vi "Build Send Method.vi"(6 "Wiring Spec":T2, 8 "error in (no error)":errorcluster, 9 "AF Library FQN":string, 10 "References":T1, 11 "Send VI":refnum<vi>) -> (0 "error out":errorcluster)   [LabVIEW 2023, in "Message Maker.lvclass"]
doc: "Build The send vi for the new message\n\nAuthor: Derek Trepanier\nCopyright: MGI 2015"
uses:
  Message Maker.lvclass
  Wiring Spec.ctl
  Connector Pane Position.ctl
  Scripting Refs.ctl
  <vilib>/Utility/traverseref.llb/TRef TravTarget.ctl
  <vilib>/Utility/miscctls.llb/LVPointTypeDef.ctl
  <vilib>/Utility/traverseref.llb/VI Scripting - Traverse.lvlib
  <vilib>/LabVIEW Icon API/LabVIEW Icon API.lvlib
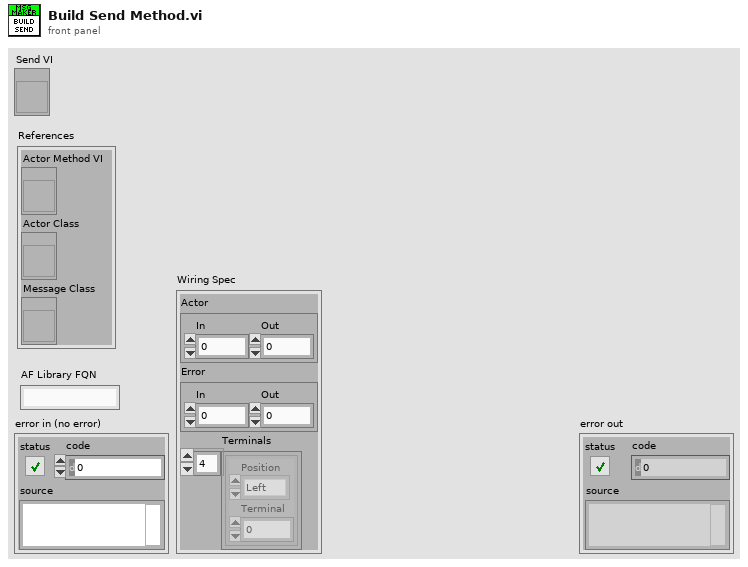
[diagram p1: front panel]
types:
  T1 = typedef "Message Maker.lvclass/Scripting Refs.ctl" = cluster{"Actor Method VI":refnum<vi>, "Actor Class":refnum<vi>, "Message Class":refnum<vi>}
  T2 = typedef "Message Maker.lvclass/Wiring Spec.ctl" = cluster{"Actor":cluster{"In":i32, "Out":i32}, "Error":cluster{"In":i32, "Out":i32}, "Terminals":cluster{"Position":T3, "Terminal":i32}[]}
  T3 = typedef "Message Maker.lvclass/Connector Pane Position.ctl" = enum16{"Left", "Top", "Bottom", "Right"}
  T4 = cluster{"Left":cluster{"Position":i16, "Index":i32}[], "Bottom":cluster{"Position":i16, "Index":i32}[], "Right":cluster{"Position":i16, "Index":i32}[], "Top":cluster{"Position":i16, "Index":i32}[]}
  T5 = enum16{"Replace Classes", "Configure Connector", "Add FP Controls", "Wire Bundle", "Set Icon and Desc", "Build BD"}
  T6 = typedef "TRef TravTarget.ctl" = enum16{"FP", "BD", "Other"}
  T7 = typedef "LVPointTypeDef.ctl" = cluster{"Horizontal":i16, "Vertical":i16}
  T8 = typedef "LVRectTypeDef.ctl" = cluster{"Left":i16, "Top":i16, "Right":i16, "Bottom":i16}
  T9 = enum16{"Invalid Wire Rule", "Required", "Recommended", "Optional", "Dynamic Dispatch"}[]
  T10 = cluster{cluster{"Position":i16, "Index":i32}[]}[]
  T11 = enum16{"Invalid Wire Rule", "Required", "Recommended", "Optional", "Dynamic Dispatch"}
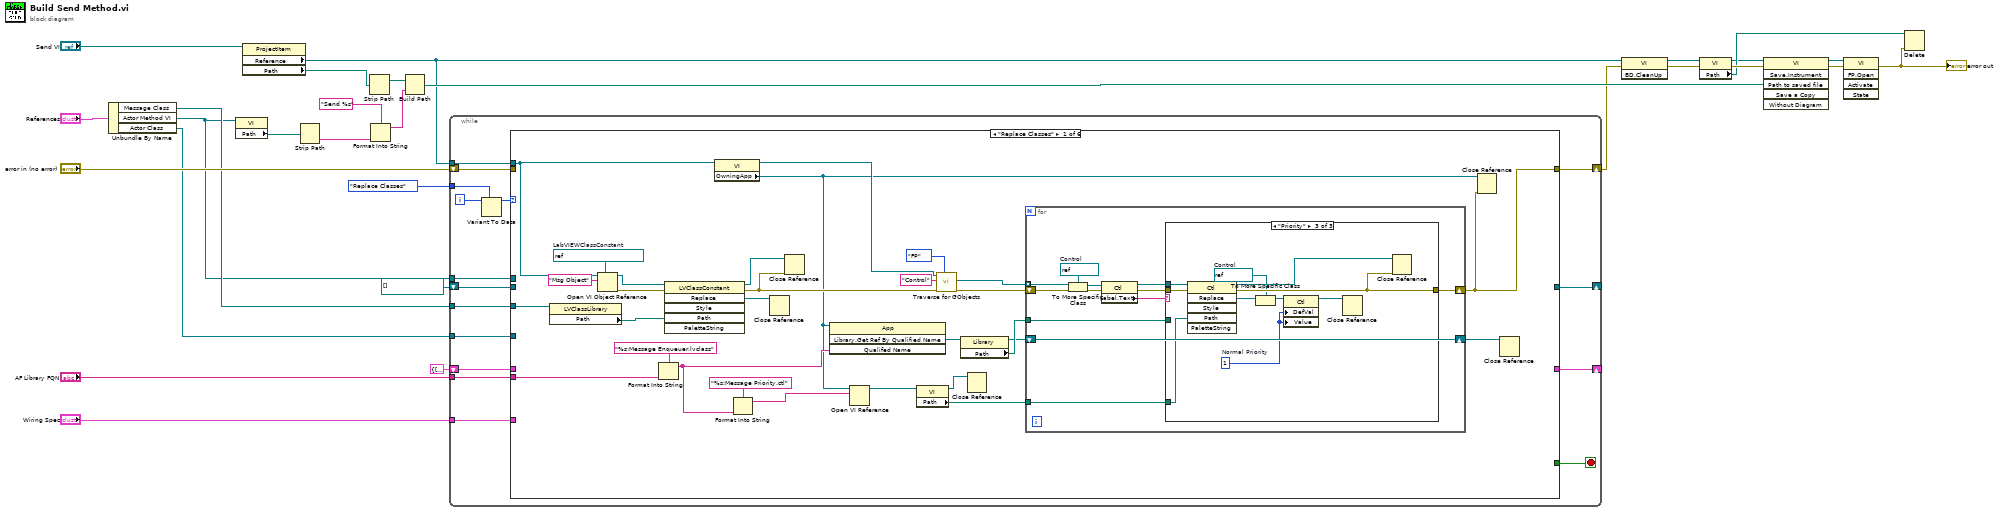
[diagram p0: block diagram]
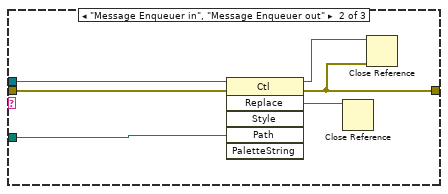
[diagram p3: hidden frame]
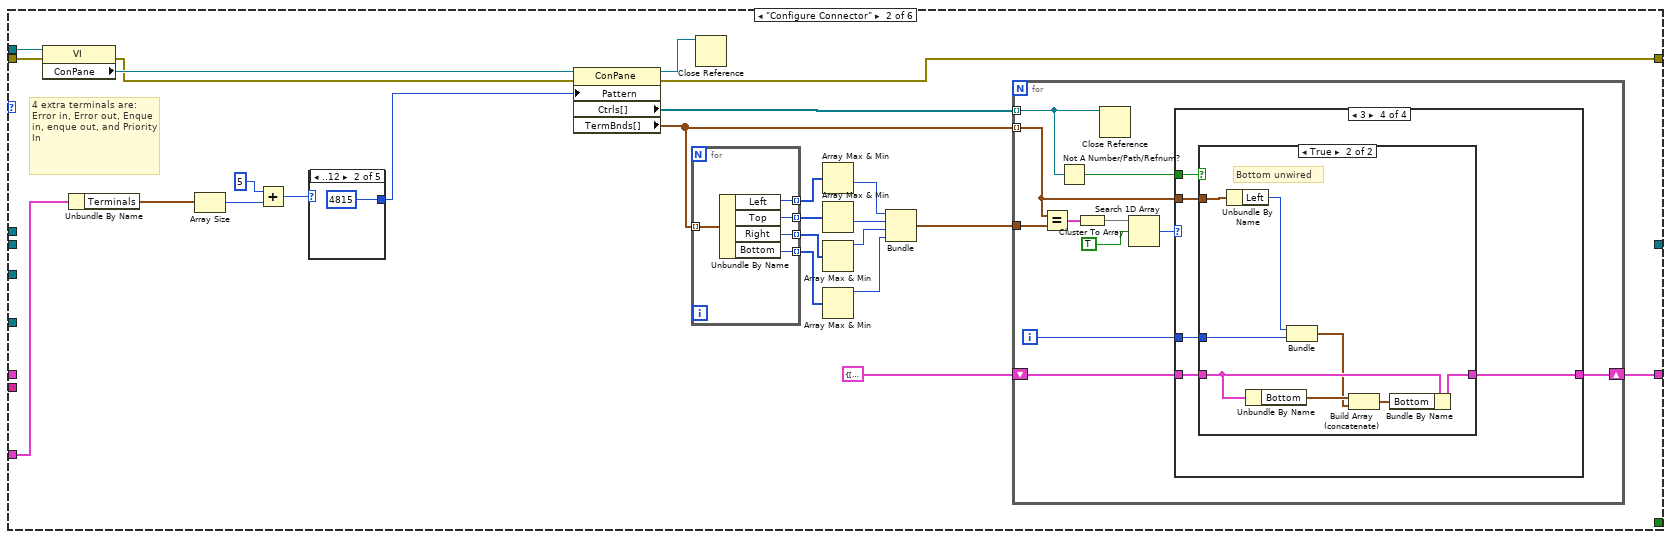
[diagram p4: hidden frame]
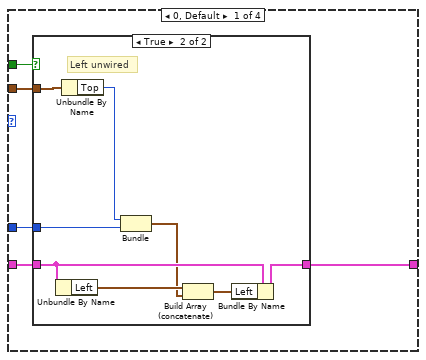
[diagram p5: hidden frame]
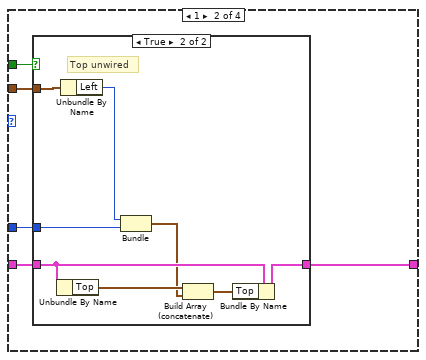
[diagram p7: hidden frame]
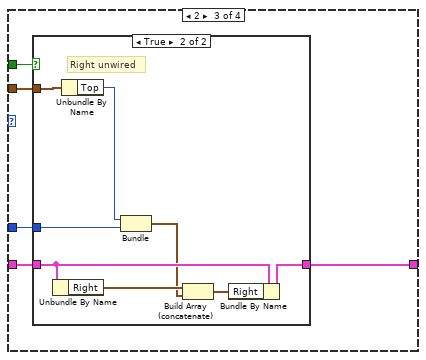
[diagram p9: hidden frame]
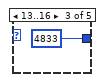
[diagram p13: hidden frame]
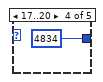
[diagram p14: hidden frame]
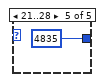
[diagram p15: hidden frame]
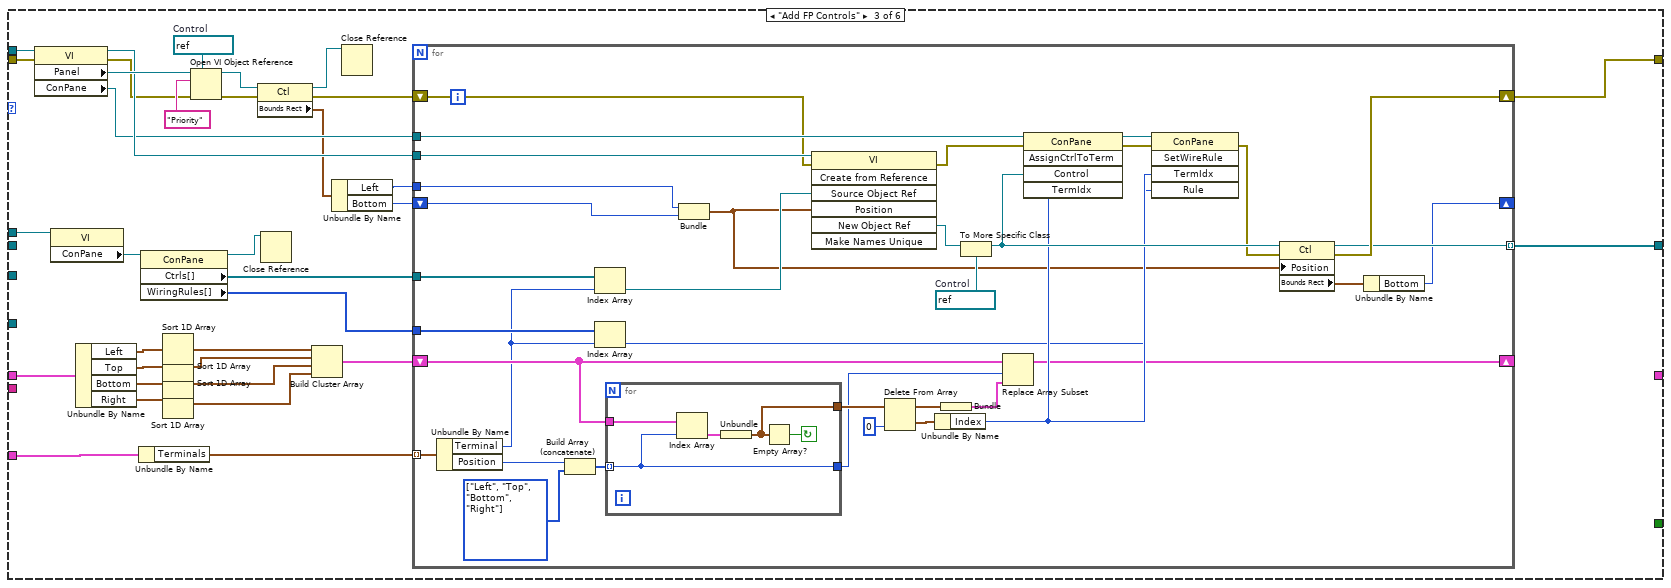
[diagram p16: hidden frame]
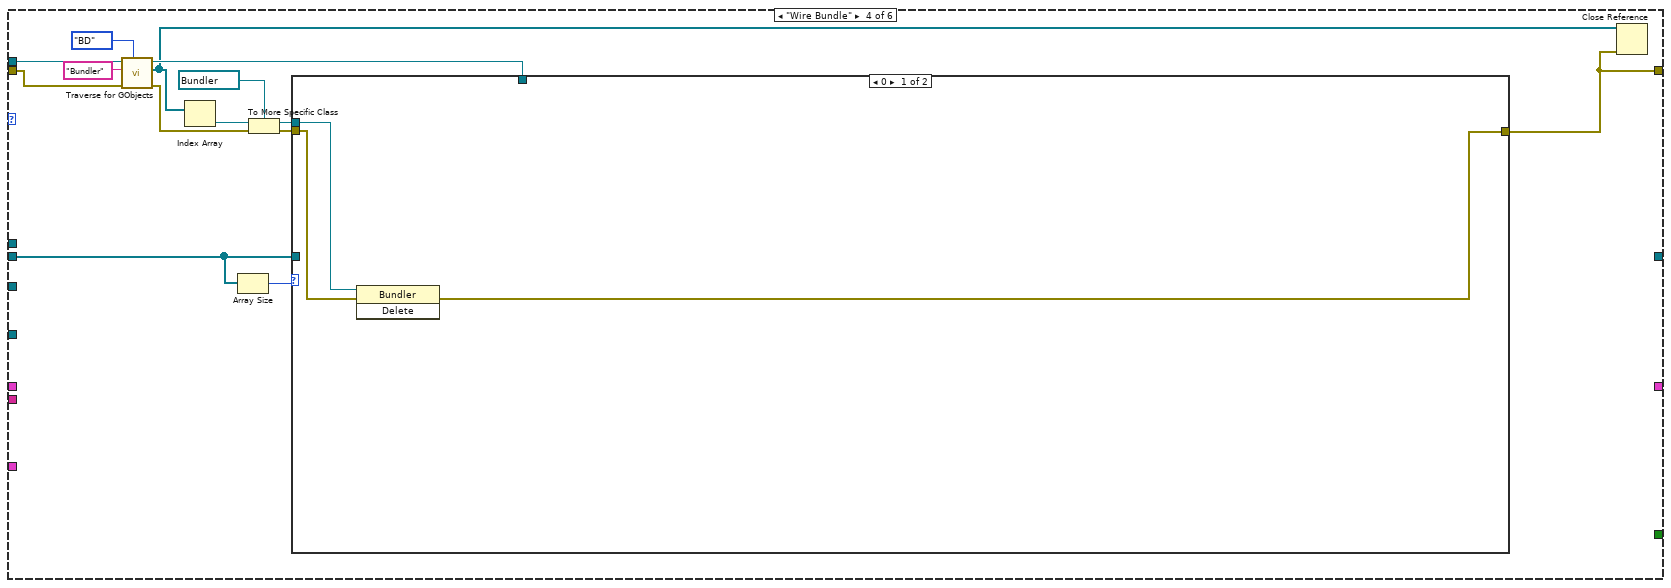
[diagram p17: hidden frame]
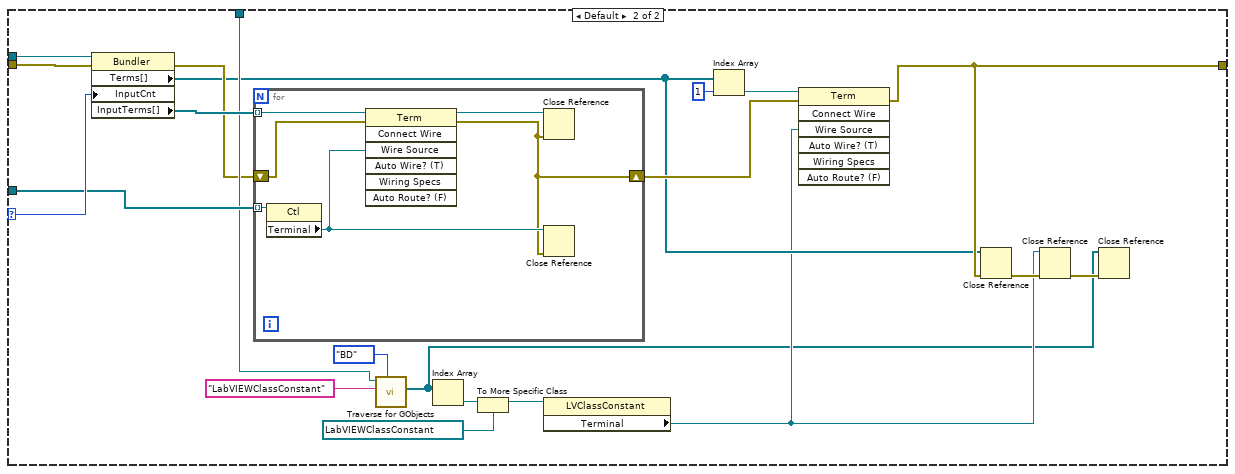
[diagram p18: hidden frame]
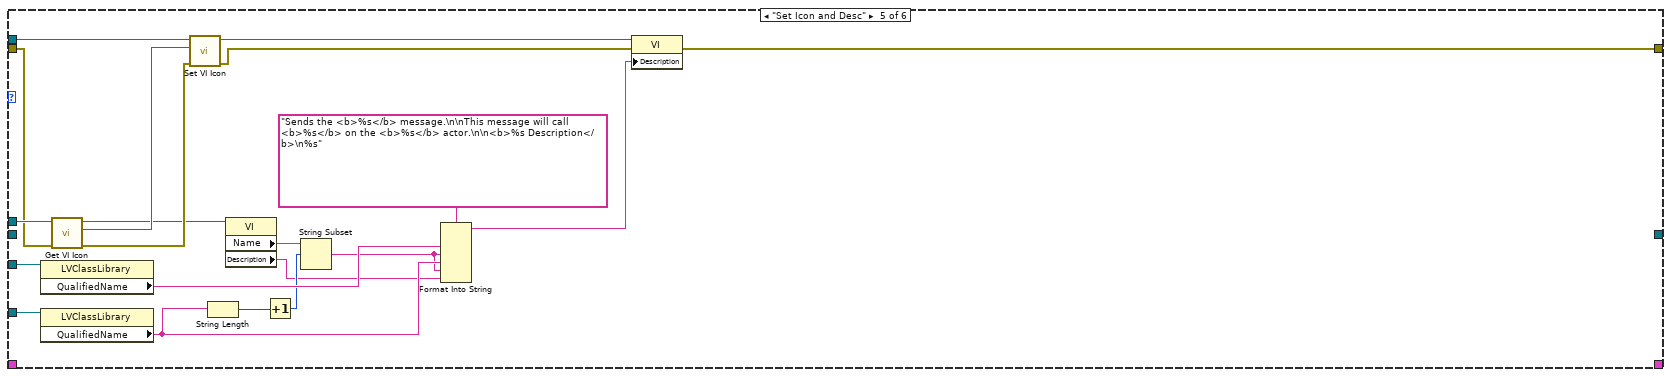
[diagram p19: hidden frame]
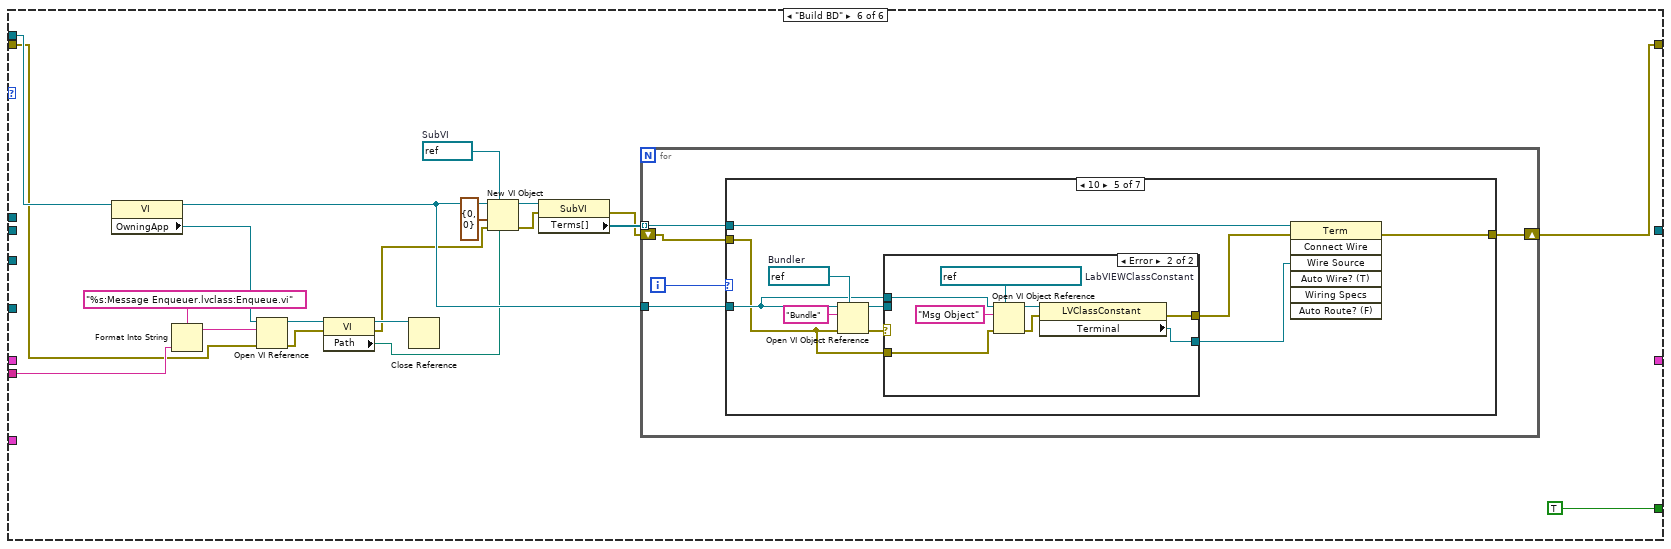
[diagram p20: hidden frame]
diagram:
  n1 = Unbundle By Name("References") -> ("Message Class"=w10:refnum<vi>, "Actor Method VI"=w5:refnum<vi>, "Actor Class"=w9:refnum<vi>)
  n2 = property class="VI"(reference=w5) -> ("Path"=w4:path)  [unwired: 1 in, 2 out]
  n3 = property class="ProjectItem"(reference="Send VI") -> ("Reference"=w19:refnum<vi>, "Path"=w25:path)  [unwired: 1 in, 2 out]
  n4 = Strip Path(path=w4) -> (name=w3:string)  [unwired: 1 out]
  n5 = Strip Path(path=w25) -> (stripped path=w24:path)  [unwired: 1 out]
  n6 = Format Into String(format string="Send %s", w3) -> (resulting string=w23:string)  [unwired: 2 in, 1 out]
  n7 = Build Path(base path=w24, name or relative path=w23) -> (appended path=w22:path)
  n8 = while {
    tunnel: T5."Replace Classes" -> [w44]
    tunnel: "Wiring Spec" -> [w41]
    tunnel: w19 -> [w40]
    tunnel: w5 -> [w39]
    shift-right: [w36] -> w17
    shift-left: "error in (no error)" -> [w37]
    shift-right: [w35] -> _
    shift-left: T4 {"Left"=[], "Bottom"=[], "Right"=[], "Top"=[]} -> [w34]
    shift-right: [w33] -> _
    shift-left: refnum<vi>[] [] -> [w32]
    tunnel: w10 -> [w31]
    tunnel: w9 -> [w30]
    tunnel: "AF Library FQN" -> [w29]
    i -> [w43]
    stop <- w38 stop-if-true
    n9 = Variant To Data(type=w44, Variant=w43) -> (data=w42:T5)  [unwired: 1 in, 1 out]
    n10 = case shown="\"Replace Classes\"" w42 {
      tunnel: w41 -> [_ w127 w228 _ _ _]
      tunnel: w40 -> [w62 w126 w237 w278 w340 w356]
      tunnel: w39 -> [_ _ w230 _ w341 _]
      tunnel: [_ _ _ _ _ TRUE] -> w38
      tunnel: w37 -> [_ w121 w223 w291 w324 w344]
      tunnel: [w46 w119 w220 w279 w322 w347] -> w36
      tunnel: [_ w103 _ _ _ _] -> w35
      tunnel: w34 -> [_ _ w219 _ _ _]
      tunnel: [_ _ w207 _ _ _] -> w33
      tunnel: w32 -> [_ _ _ w286 _ _]
      tunnel: w31 -> [w71 _ _ _ w333 _]
      tunnel: w30 -> [_ _ _ _ w331 _]
      tunnel: w29 -> [w48 _ _ _ _ w349]
      frame "Replace Classes" {
        w68 = refnum<vi> refnum  # LabVIEWClassConstant
        n11 = property class="LVClassLibrary"(reference=w71) -> ("Path"=w73:path)  [unwired: 1 in, 2 out]
        n12 = Open VI Object Reference(7:w68, 10:"Msg Object" ("name/order"), 11:w62) -> (0:w70:errorcluster, 3:w69:refnum<vi>)  [unwired: 1 in]
        n13 = Format Into String(format string="%s:Message Enqueuer.lvclass", w48) -> (resulting string=w49:string)  [unwired: 2 in, 1 out]
        n14 = invoke class="LVClassConstant" method="Replace"(reference=w69, error in=w70, "Path"=w73) -> (reference out=w67:refnum<vi>, error out=w63:errorcluster, "Replace"=w72:refnum<vi>)  [unwired: 3 in, 3 out]
        n15 = property class="VI"(reference=w62) -> (reference out=w59:refnum<vi>, "OwningApp"=w45:refnum<vi>)  [unwired: 1 in, 1 out]
        n16 = Format Into String(format string="%s:Message Priority.ctl", w49) -> (resulting string=w53:string)  [unwired: 2 in, 1 out]
        n17 = Close Reference(reference=w72) -> ()  [unwired: 1 in, 1 out]
        n18 = Close Reference(reference=w67, error in (no error)=w63) -> ()  [unwired: 1 out]
        n19 = invoke class="App" method="Library.Get Ref By Qualified Name"(reference=w45, "Qualifed Name"=w49) -> ("Library.Get Ref By Qualified Name"=w58:refnum<vi>)  [unwired: 2 in, 3 out]
        n20 = Open VI Reference(application reference (local)=w45, vi path=w53) -> (vi reference=w52:refnum<vi>)  [unwired: 4 in, 1 out]
        n21 = property class="VI"(reference=w52) -> (reference out=w47:refnum<vi>, "Path"=w51:path)  [unwired: 1 in, 1 out]
        n22 = call <vilib>:"Traverse for GObjects.vi"("Traverse Target"=TRef_TravTarget."FP", "error in (no error)"=w63, "Class Name"="Control" ("name/order"), "VI Refnum"=w59) -> ("error out"=w64:errorcluster, "References"=w60:refnum<vi>[])  [unwired: 4 in, 2 out]
        n23 = property class="Library"(reference=w58) -> (reference out=w56:refnum<vi>, "Path"=w57:path)  [unwired: 1 in, 1 out]
        n24 = Close Reference(reference=w47) -> ()  [unwired: 1 in, 1 out]
        n25 = for {
          tunnel: w60 -> [w78] mode=indexing
          tunnel: w57 -> [w84]
          shift-right: [w83] -> w46
          shift-left: w64 -> [w85]
          shift-right: [w82] -> w55
          shift-left: w56 -> [w82]
          tunnel: w51 -> [w74]
          w76 = refnum<vi> refnum  # Control
          n26 = To More Specific Class(target class=w76, reference=w78, error in=w85) -> (specific class reference=w77:refnum<vi>, error out=w79:errorcluster)
          n27 = property class="Ctl"(reference=w77, error in=w79) -> (reference out=w80:refnum<vi>, error out=w81:errorcluster, "Label.Text"=w75:string)
          n28 = case shown="\"Priority\"" w75 {
            tunnel: w84 -> [_ w90 _]
            tunnel: [w86 w89 w100] -> w83
            tunnel: w81 -> [w86 w88 w99]
            tunnel: w80 -> [_ w87 w98]
            tunnel: w74 -> [_ _ w97]
            frame "False", Default {
            }
            frame "Message Enqueuer in", "Message Enqueuer out" {
              n29 = invoke class="Ctl" method="Replace"(reference=w87, error in=w88, "Path"=w90) -> (reference out=w92:refnum<vi>, error out=w89:errorcluster, "Replace"=w91:refnum<vi>)  [unwired: 3 in, 3 out]
              n30 = Close Reference(reference=w91) -> ()  [unwired: 1 in, 1 out]
              n31 = Close Reference(reference=w92, error in (no error)=w89) -> ()  [unwired: 1 out]
            }
            frame "Priority" {
              w93 = 1  # Normal Priority
              w94 = refnum<vi> refnum  # Control
              n32 = invoke class="Ctl" method="Replace"(reference=w98, error in=w99, "Path"=w97) -> (reference out=w102:refnum<vi>, error out=w100:errorcluster, "Replace"=w101:refnum<vi>)  [unwired: 3 in, 3 out]
              n33 = To More Specific Class(target class=w94, reference=w101) -> (specific class reference=w95:refnum<vi>)  [unwired: 1 in, 1 out]
              n34 = property class="Ctl"(reference=w95, "DefVal"=w93, "Value"=w93) -> (reference out=w96:refnum<vi>)  [unwired: 1 in, 1 out]
              n35 = Close Reference(reference=w96) -> ()  [unwired: 1 in, 1 out]
              n36 = Close Reference(reference=w102, error in (no error)=w100) -> ()  [unwired: 1 out]
            }
          }
        }
        n37 = Close Reference(reference=w45, error in (no error)=w46) -> ()  [unwired: 1 out]
        n38 = Close Reference(reference=w55) -> ()  [unwired: 1 in, 1 out]
      }
      frame "Configure Connector" {
        # "4 extra terminals are:\nError in, Error out, Enque in, enque out, and Priority In"
        n39 = property class="VI"(reference=w126, error in=w121) -> (error out=w120:errorcluster, "ConPane"=w125:refnum<vi>)  [unwired: 1 out]
        n40 = Unbundle By Name(w127) -> ("Terminals"=w124:cluster{"Position":T3, "Terminal":i32}[])
        n41 = Array Size(array=w124) -> (size(s)=w118:i32)
        n42 = Add(x=5, y=w118) -> (x+y=w116:i32)
        n43 = case shown="..12" w116 {
          tunnel: [_ u32 4815 ("Pattern") u32 4833 ("Pattern") u32 4834 ("Pattern") u32 4835 ("Pattern")] -> w122
          frame Default {
          }
          frame ..12 {
          }
          frame 13..16 {
          }
          frame 17..20 {
          }
          frame 21..28 {
          }
        }
        n44 = property class="ConPane"(reference=w125, error in=w120, "Pattern"=w122) -> (reference out=w123:refnum<vi>, error out=w119:errorcluster, "Ctrls[]"=w109:refnum<vi>[], "TermBnds[]"=w107:T8[])
        n45 = for {
          tunnel: w107 -> [w199] mode=indexing
          tunnel: [w198] -> w115 mode=indexing
          tunnel: [w197] -> w114 mode=indexing
          tunnel: [w196] -> w113 mode=indexing
          tunnel: [w195] -> w112 mode=indexing
          n46 = Unbundle By Name(w199) -> ("Left"=w198:i16, "Top"=w197:i16, "Right"=w196:i16, "Bottom"=w195:i16)
        }
        n47 = Close Reference(reference=w123) -> ()  [unwired: 1 in, 1 out]
        n48 = Array Max & Min(array=w115) -> (min value=w106:i16)  [unwired: 3 out]
        n49 = Array Max & Min(array=w114) -> (min value=w105:i16)  [unwired: 3 out]
        n50 = Array Max & Min(array=w113) -> (max value=w111:i16)  [unwired: 3 out]
        n51 = Array Max & Min(array=w112) -> (max value=w110:i16)  [unwired: 3 out]
        n52 = Bundle(w106, w105, w111, w110) -> (w108:cluster{i16, i16, i16, i16})  [unwired: 1 in]
        n53 = for {
          tunnel: w109 -> [w133] mode=indexing
          tunnel: w108 -> [w138]
          tunnel: w107 -> [w130] mode=indexing
          shift-right: [w129] -> w103
          shift-left: T4 {"Left"=[], "Bottom"=[], "Right"=[], "Top"=[]} -> [w131]
          i -> [w128]
          n54 = Equal?(x=w130, y=w138) -> (x = y?=w137:cluster{bool, bool, bool, bool})
          n55 = Not A Number/Path/Refnum?(number/path/refnum=w133) -> (NaN/Path/Refnum?=w132:bool)
          n56 = Cluster To Array(cluster=w137) -> (array=w136:bool[])
          n57 = Close Reference(reference=w133) -> ()  [unwired: 1 in, 1 out]
          n58 = Search 1D Array(1D array=w136, element=TRUE) -> (index of element=w134:i32)  [unwired: 1 in]
          n59 = case shown="3" w134 {
            tunnel: w132 -> [w143 w157 w171 w185]
            tunnel: w131 -> [w142 w156 w170 w184]
            tunnel: w130 -> [w141 w155 w169 w183]
            tunnel: [w140 w154 w168 w182] -> w129
            tunnel: w128 -> [w139 w153 w167 w181]
            frame 0, Default {
              n60 = case shown="True" w143 {
                tunnel: w142 -> [w144 w151]
                tunnel: w141 -> [_ w152]
                tunnel: [w144 w148] -> w140
                tunnel: w139 -> [_ w149]
                frame False {
                }
                frame True {
                  # "Left unwired"
                  n61 = Unbundle By Name(w151) -> ("Left"=w147:cluster{"Position":i16, "Index":i32}[])
                  n62 = Unbundle By Name(w152) -> ("Top"=w150:i16)
                  n63 = Bundle("Top"=w150, w149) -> (w145:cluster{"Top":i16, i32})  [unwired: 1 in]
                  n64 = Build Array (concatenate)(w147, w145) -> (w146:cluster{"Top":i16, "Index":i32}[])
                  n65 = Bundle By Name(cluster=w151, "Left"=w146) -> (w148:T4)
                }
              }
            }
            frame 1 {
              n66 = case shown="True" w157 {
                tunnel: w156 -> [w158 w165]
                tunnel: w155 -> [_ w166]
                tunnel: [w158 w162] -> w154
                tunnel: w153 -> [_ w163]
                frame False {
                }
                frame True {
                  # "Top unwired"
                  n67 = Unbundle By Name(w165) -> ("Top"=w161:cluster{"Position":i16, "Index":i32}[])
                  n68 = Unbundle By Name(w166) -> ("Left"=w164:i16)
                  n69 = Bundle("Left"=w164, w163) -> (w159:cluster{"Left":i16, i32})  [unwired: 1 in]
                  n70 = Build Array (concatenate)(w161, w159) -> (w160:cluster{"Left":i16, "Index":i32}[])
                  n71 = Bundle By Name(cluster=w165, "Top"=w160) -> (w162:T4)
                }
              }
            }
            frame 2 {
              n72 = case shown="True" w171 {
                tunnel: w170 -> [w172 w179]
                tunnel: w169 -> [_ w180]
                tunnel: [w172 w176] -> w168
                tunnel: w167 -> [_ w177]
                frame False {
                }
                frame True {
                  # "Right unwired"
                  n73 = Unbundle By Name(w179) -> ("Right"=w175:cluster{"Position":i16, "Index":i32}[])
                  n74 = Unbundle By Name(w180) -> ("Top"=w178:i16)
                  n75 = Bundle("Top"=w178, w177) -> (w173:cluster{"Top":i16, i32})  [unwired: 1 in]
                  n76 = Build Array (concatenate)(w175, w173) -> (w174:cluster{"Top":i16, "Index":i32}[])
                  n77 = Bundle By Name(cluster=w179, "Right"=w174) -> (w176:T4)
                }
              }
            }
            frame 3 {
              n78 = case shown="True" w185 {
                tunnel: w184 -> [w186 w193]
                tunnel: w183 -> [_ w194]
                tunnel: [w186 w190] -> w182
                tunnel: w181 -> [_ w191]
                frame False {
                }
                frame True {
                  # "Bottom unwired"
                  n79 = Unbundle By Name(w194) -> ("Left"=w192:i16)
                  n80 = Unbundle By Name(w193) -> ("Bottom"=w189:cluster{"Position":i16, "Index":i32}[])
                  n81 = Bundle("Left"=w192, w191) -> (w187:cluster{"Left":i16, i32})  [unwired: 1 in]
                  n82 = Build Array (concatenate)(w189, w187) -> (w188:cluster{"Left":i16, "Index":i32}[])
                  n83 = Bundle By Name(cluster=w193, "Bottom"=w188) -> (w190:T4)
                }
              }
            }
          }
        }
      }
      frame "Add FP Controls" {
        w236 = refnum<vi> refnum  # Control
        n84 = property class="VI"(reference=w237, error in=w223) -> (reference out=w225:refnum<vi>, error out=w222:errorcluster, "Panel"=w234:refnum<vi>, "ConPane"=w224:refnum<vi>)
        n85 = property class="VI"(reference=w230) -> ("ConPane"=w229:refnum<vi>)  [unwired: 1 in, 2 out]
        n86 = Unbundle By Name(w219) -> ("Left"=w218:cluster{"Position":i16, "Index":i32}[], "Top"=w217:cluster{"Position":i16, "Index":i32}[], "Bottom"=w215:cluster{"Position":i16, "Index":i32}[], "Right"=w216:cluster{"Position":i16, "Index":i32}[])
        n87 = Unbundle By Name(w228) -> ("Terminals"=w226:cluster{"Position":T3, "Terminal":i32}[])
        n88 = property class="ConPane"(reference=w229) -> (reference out=w209:refnum<vi>, "Ctrls[]"=w227:refnum<vi>[], "WiringRules[]"=w210:T9)  [unwired: 1 in, 1 out]
        n89 = Sort 1D Array(array=w218) -> (sorted array=w214:cluster{"Position":i16, "Index":i32}[])
        n90 = Sort 1D Array(array=w217) -> (sorted array=w208:cluster{"Position":i16, "Index":i32}[])
        n91 = Sort 1D Array(array=w215) -> (sorted array=w213:cluster{"Position":i16, "Index":i32}[])
        n92 = Sort 1D Array(array=w216) -> (sorted array=w212:cluster{"Position":i16, "Index":i32}[])
        n93 = Open VI Object Reference(7:w236, 8:w222, 10:"Priority" ("name/order"), 11:w234) -> (0:w231:errorcluster, 3:w233:refnum<vi>)
        n94 = property class="Ctl"(reference=w233, error in=w231) -> (reference out=w232:refnum<vi>, error out=w221:errorcluster, "Bounds Rect"=w206:T8)
        n95 = Close Reference(reference=w209) -> ()  [unwired: 1 in, 1 out]
        n96 = Build Cluster Array(w214, w208, w213, w212) -> (w211:T10)
        n97 = Unbundle By Name(w206) -> ("Left"=w205:i16, "Bottom"=w204:i16)
        n98 = Close Reference(reference=w232) -> ()  [unwired: 1 in, 1 out]
        n99 = for {
          tunnel: w227 -> [w272]
          tunnel: w226 -> [w264] mode=indexing
          tunnel: w225 -> [w271]
          tunnel: w224 -> [w270]
          shift-right: [w265] -> w220
          shift-left: w221 -> [w267]
          shift-right: [w249] -> _
          shift-left: w211 -> [w257]
          tunnel: w210 -> [w248]
          tunnel: [w245] -> w207 mode=indexing
          tunnel: w205 -> [w239]
          shift-right: [w240] -> _
          shift-left: w204 -> [w238]
          w262 = T3[] [enum."Left", enum."Top", enum."Bottom", enum."Right"] items=["Left", "Top", "Bottom", "Right"] ("appended array")
          w269 = refnum<vi> refnum  # Control
          n100 = Unbundle By Name(w264) -> ("Terminal"=w246:i32, "Position"=w263:T3)
          n101 = Build Array (concatenate)(w263, w262) -> (w261:T3[])
          n102 = Index Array(array=w272, index=w246) -> (element=w243:refnum<vi>)
          n103 = Index Array(array=w248, index=w246) -> (element=w247:T11)
          n104 = for {
            tunnel: w257 -> [w277]
            tunnel: w261 -> [w274] mode=indexing
            tunnel: [w274] -> w255
            tunnel: [w273] -> w260
            stop <- w275 continue-if-true
            n105 = Index Array(array=w277, index=w274) -> (element=w276:cluster{cluster{"Position":i16, "Index":i32}[]})
            n106 = Unbundle(w276) -> (w273:cluster{"Position":i16, "Index":i32}[])
            n107 = Empty Array?(array=w273) -> (empty?=w275:bool)
          }
          n108 = Bundle("Left"=w239, "Bottom"=w238) -> (w242:cluster{"Left":i16, "Bottom":i16})  [unwired: 1 in]
          n109 = invoke class="VI" method="Create from Reference"(reference=w271, error in=w267, "Source Object Ref"=w243, "Position"=w242) -> (error out=w266:errorcluster, "New Object Ref"=w244:refnum<vi>)  [unwired: 3 in, 5 out]
          n110 = Delete From Array(array=w260, index=0) -> (deleted portion=w254:cluster{"Position":i16, "Index":i32}, array with subset deleted=w258:cluster{"Position":i16, "Index":i32}[])  [unwired: 1 in]
          n111 = Unbundle By Name(w254) -> ("Index"=w250:i32)
          n112 = Bundle(w258) -> (w256:cluster{cluster{"Position":i16, "Index":i32}[]})  [unwired: 1 in]
          n113 = To More Specific Class(target class=w269, reference=w244) -> (specific class reference=w268:refnum<vi>)  [unwired: 1 in, 1 out]
          n114 = Replace Array Subset(array=w257, new element=w256, index=w255) -> (w249:T10)
          n115 = invoke class="ConPane" method="AssignCtrlToTerm"(reference=w270, error in=w266, "Control"=w268, "TermIdx"=w250) -> (reference out=w253:refnum<vi>, error out=w252:errorcluster)  [unwired: 1 in, 3 out]
          n116 = invoke class="ConPane" method="SetWireRule"(reference=w253, error in=w252, "TermIdx"=w250, "Rule"=w247) -> (error out=w251:errorcluster)  [unwired: 1 in, 4 out]
          n117 = property class="Ctl"(reference=w268, error in=w251, "Position"=w242) -> (reference out=w245:refnum<vi>, error out=w265:errorcluster, "Bounds Rect"=w241:T8)
          n118 = Unbundle By Name(w241) -> ("Bottom"=w240:i16)
        }
      }
      frame "Wire Bundle" {
        n119 = call <vilib>:"Traverse for GObjects.vi"("Traverse Target"=TRef_TravTarget."BD", "error in (no error)"=w291, "Class Name"="Bundler", "VI Refnum"=w278) -> ("error out"=w283:errorcluster, "References"=w280:refnum<vi>[], "dup VI Refnum"=w281:refnum<vi>)  [unwired: 4 in, 1 out]
        n120 = Index Array(array=w280) -> (element=w288:refnum<vi>)  [unwired: 1 in]
        n121 = Array Size(array=w286) -> (size(s)=w285:i32)
        n122 = To More Specific Class(target class=refnum<vi> refnum ("element"), reference=w288, error in=w283) -> (specific class reference=w284:refnum<vi>, error out=w282:errorcluster)
        n123 = case shown="0" w285 {
          selector: w285 -> [_ w313]
          tunnel: w286 -> [_ w311]
          tunnel: w284 -> [w294 w315]
          tunnel: w282 -> [w293 w314]
          tunnel: w281 -> [_ w308]
          tunnel: [w292 w300] -> w279
          frame 0 {
            n124 = invoke class="Bundler" method="Delete"(reference=w294, error in=w293) -> (error out=w292:errorcluster)  [unwired: 1 in, 2 out]
          }
          frame Default {
            n125 = property class="Bundler"(reference=w315, error in=w314, "InputCnt"=w313) -> (error out=w302:errorcluster, "Terms[]"=w299:refnum<vi>[], "InputTerms[]"=w312:refnum<vi>[])  [unwired: 1 out]
            n126 = for {
              tunnel: w312 -> [w321] mode=indexing
              tunnel: w311 -> [w319] mode=indexing
              shift-right: [w317] -> w303
              shift-left: w302 -> [w316]
              n127 = property class="Ctl"(reference=w319) -> ("Terminal"=w318:refnum<vi>)  [unwired: 1 in, 2 out]
              n128 = invoke class="Term" method="Connect Wire"(reference=w321, error in=w316, "Wire Source"=w318) -> (reference out=w320:refnum<vi>, error out=w317:errorcluster)  [unwired: 4 in, 5 out]
              n129 = Close Reference(reference=w320, error in (no error)=w317) -> ()  [unwired: 1 out]
              n130 = Close Reference(reference=w318, error in (no error)=w317) -> ()  [unwired: 1 out]
            }
            n131 = call <vilib>:"Traverse for GObjects.vi"("Traverse Target"=TRef_TravTarget."BD", "Class Name"="LabVIEWClassConstant", "VI Refnum"=w308) -> ("References"=w295:refnum<vi>[])  [unwired: 5 in, 3 out]
            n132 = Index Array(array=w295) -> (element=w306:refnum<vi>)  [unwired: 1 in]
            n133 = To More Specific Class(target class=refnum<vi> refnum ("element"), reference=w306) -> (specific class reference=w305:refnum<vi>)  [unwired: 1 in, 1 out]
            n134 = property class="LVClassConstant"(reference=w305) -> ("Terminal"=w297:refnum<vi>)  [unwired: 1 in, 2 out]
            n135 = Index Array(array=w299, index=1) -> (element=w304:refnum<vi>)
            n136 = invoke class="Term" method="Connect Wire"(reference=w304, error in=w303, "Wire Source"=w297) -> (error out=w300:errorcluster)  [unwired: 4 in, 6 out]
            n137 = Close Reference(reference=w299, error in (no error)=w300) -> (error out=w298:errorcluster)
            n138 = Close Reference(reference=w297, error in (no error)=w298) -> (error out=w296:errorcluster)
            n139 = Close Reference(reference=w295, error in (no error)=w296) -> ()  [unwired: 1 out]
          }
        }
        n140 = Close Reference(reference=w280, error in (no error)=w279) -> ()  [unwired: 1 out]
      }
      frame "Set Icon and Desc" {
        n141 = property class="LVClassLibrary"(reference=w333) -> ("QualifiedName"=w332:string)  [unwired: 1 in, 2 out]
        n142 = property class="LVClassLibrary"(reference=w331) -> ("QualifiedName"=w327:string)  [unwired: 1 in, 2 out]
        n143 = call <vilib>:"Get VI Icon.vi"("error in (no error)"=w324, "VI Refnum in"=w341) -> ("error out"=w338:errorcluster, "Icon"=w339:refnum<class "Icon.lvclass">, "VI Refnum out"=w337:refnum<vi>)  [unwired: 7 in]
        n144 = call <vilib>:"Set VI Icon.vi"("error in (no error)"=w338, "Icon"=w339, "VI Refnum in"=w340) -> ("error out"=w323:errorcluster, "VI Refnum out"=w335:refnum<vi>)  [unwired: 7 in]
        n145 = String Length(string=w327) -> (length=w330:i32)
        n146 = property class="VI"(reference=w337) -> ("Name"=w329:string, "Description"=w325:string)  [unwired: 1 in, 2 out]
        n147 = Increment(x=w330) -> (x+1=w328:i32)
        n148 = String Subset(string=w329, offset (0)=w328) -> (substring=w326:string)  [unwired: 1 in]
        n149 = Format Into String(format string="Sends the <b>%s</b> message.\n\nThis message will call <b>%s</b> on the <b>%s</b> actor.\n\n<b>%s Description</b>\n%s", w332, w326, w327, w326, w325) -> (resulting string=w334:string)  [unwired: 2 in, 1 out]
        n150 = property class="VI"(reference=w335, error in=w323, "Description"=w334) -> (error out=w322:errorcluster)  [unwired: 1 out]
      }
      frame "Build BD" {
        w360 = refnum<vi> refnum  # SubVI
        n151 = property class="VI"(reference=w356) -> (reference out=w355:refnum<vi>, "OwningApp"=w354:refnum<vi>)  [unwired: 1 in, 1 out]
        n152 = Format Into String(format string="%s:Message Enqueuer.lvclass:Enqueue.vi", w349) -> (resulting string=w348:string)  [unwired: 2 in, 1 out]
        n153 = Open VI Reference(application reference (local)=w354, vi path=w348, error in (no error)=w344) -> (vi reference=w353:refnum<vi>, error out=w343:errorcluster)  [unwired: 3 in]
        n154 = property class="VI"(reference=w353, error in=w343) -> (reference out=w352:refnum<vi>, error out=w342:errorcluster, "Path"=w351:path)
        n155 = Close Reference(reference=w352) -> ()  [unwired: 1 in, 1 out]
        n156 = New VI Object(vi object class=w360, owner refnum=w355, position/next to=T7 {"Horizontal"=0, "Vertical"=0} ("location"), 6:w351, 8:w342) -> (object refnum=w358:refnum<vi>, 0:w345:errorcluster)  [unwired: 3 in]
        n157 = property class="SubVI"(reference=w358, error in=w345) -> (error out=w346:errorcluster, "Terms[]"=w357:refnum<vi>[])  [unwired: 1 out]
        n158 = for {
          tunnel: w357 -> [w365] mode=indexing
          tunnel: w355 -> [w364]
          shift-right: [w363] -> w347
          shift-left: w346 -> [w362]
          i -> [w366]
          n159 = case shown="10" w366 {
            tunnel: w365 -> [w376 w386 w396 w406 w416 w440 _]
            tunnel: w364 -> [w375 w385 w395 w405 w410 w439 _]
            tunnel: [w367 w377 w387 w397 w408 w431 w441] -> w363
            tunnel: w362 -> [w370 w380 w390 w400 w407 w434 w441]
            frame 0 {
              w373 = refnum<vi> refnum  # Control
              n160 = Open VI Object Reference(7:w373, 8:w370, 10:"error out" ("name/order"), 11:w375) -> (0:w369:errorcluster, 3:w372:refnum<vi>)
              n161 = property class="Ctl"(reference=w372, error in=w369) -> (error out=w368:errorcluster, "Terminal"=w371:refnum<vi>)  [unwired: 1 out]
              n162 = invoke class="Term" method="Connect Wire"(reference=w376, error in=w368, "Wire Source"=w371) -> (error out=w367:errorcluster)  [unwired: 4 in, 6 out]
            }
            frame 3 {
              w383 = refnum<vi> refnum  # Control
              n163 = Open VI Object Reference(7:w383, 8:w380, 10:"Message Enqueuer out" ("name/order"), 11:w385) -> (0:w379:errorcluster, 3:w382:refnum<vi>)
              n164 = property class="Ctl"(reference=w382, error in=w379) -> (error out=w378:errorcluster, "Terminal"=w381:refnum<vi>)  [unwired: 1 out]
              n165 = invoke class="Term" method="Connect Wire"(reference=w386, error in=w378, "Wire Source"=w381) -> (error out=w377:errorcluster)  [unwired: 4 in, 6 out]
            }
            frame 8 {
              w393 = refnum<vi> refnum  # Control
              n166 = Open VI Object Reference(7:w393, 8:w390, 10:"error in (no error)" ("name/order"), 11:w395) -> (0:w389:errorcluster, 3:w392:refnum<vi>)
              n167 = property class="Ctl"(reference=w392, error in=w389) -> (error out=w388:errorcluster, "Terminal"=w391:refnum<vi>)  [unwired: 1 out]
              n168 = invoke class="Term" method="Connect Wire"(reference=w396, error in=w388, "Wire Source"=w391) -> (error out=w387:errorcluster)  [unwired: 4 in, 6 out]
            }
            frame 9 {
              w403 = refnum<vi> refnum  # Control
              n169 = Open VI Object Reference(7:w403, 8:w400, 10:"Priority" ("name/order"), 11:w405) -> (0:w399:errorcluster, 3:w402:refnum<vi>)
              n170 = property class="Ctl"(reference=w402, error in=w399) -> (error out=w398:errorcluster, "Terminal"=w401:refnum<vi>)  [unwired: 1 out]
              n171 = invoke class="Term" method="Connect Wire"(reference=w406, error in=w398, "Wire Source"=w401) -> (error out=w397:errorcluster)  [unwired: 4 in, 6 out]
            }
            frame 10 {
              w414 = refnum<vi> refnum  # Bundler
              n172 = Open VI Object Reference(7:w414, 8:w407, 10:"Bundle" ("name/order"), 11:w410) -> (0:w411:errorcluster, 3:w413:refnum<vi>)
              n173 = case shown="Error" w411 {
                selector: w411 -> [w418 _]
                tunnel: w413 -> [w422 _]
                tunnel: [w420 w425] -> w412
                tunnel: w410 -> [_ w428]
                tunnel: [w417 w424] -> w409
                tunnel: w407 -> [_ w423]
                frame No Error {
                  n174 = property class="Bundler"(reference=w422, error in=w418, "Label.Visible"=FALSE) -> (error out=w417:errorcluster, "Terms[]"=w421:refnum<vi>[])  [unwired: 1 out]
                  n175 = Index Array(array=w421) -> (element=w420:refnum<vi>)  [unwired: 1 in]
                }
                frame Error {
                  w430 = refnum<vi> refnum  # LabVIEWClassConstant
                  n176 = Open VI Object Reference(7:w430, 8:w423, 10:"Msg Object" ("name/order"), 11:w428) -> (0:w426:errorcluster, 3:w427:refnum<vi>)
                  n177 = property class="LVClassConstant"(reference=w427, error in=w426) -> (error out=w424:errorcluster, "Terminal"=w425:refnum<vi>)  [unwired: 1 out]
                }
              }
              n178 = invoke class="Term" method="Connect Wire"(reference=w416, error in=w409, "Wire Source"=w412) -> (error out=w408:errorcluster)  [unwired: 4 in, 6 out]
            }
            frame 11 {
              w437 = refnum<vi> refnum  # Control
              n179 = Open VI Object Reference(7:w437, 8:w434, 10:"Message Enqueuer in" ("name/order"), 11:w439) -> (0:w433:errorcluster, 3:w436:refnum<vi>)
              n180 = property class="Ctl"(reference=w436, error in=w433) -> (error out=w432:errorcluster, "Terminal"=w435:refnum<vi>)  [unwired: 1 out]
              n181 = invoke class="Term" method="Connect Wire"(reference=w440, error in=w432, "Wire Source"=w435) -> (error out=w431:errorcluster)  [unwired: 4 in, 6 out]
            }
            frame Default {
            }
          }
        }
      }
    }
  }
  n182 = invoke class="VI" method="BD.CleanUp"(reference=w19, error in=w17) -> (reference out=w26:refnum<vi>, error out=w13:errorcluster)  [unwired: 1 in, 1 out]
  n183 = property class="VI"(reference=w26, error in=w13) -> (reference out=w2:refnum<vi>, error out=w14:errorcluster, "Path"=w12:path)
  n184 = invoke class="VI" method="Save.Instrument"(reference=w2, error in=w14, "Path to saved file"=w22) -> (reference out=w8:refnum<vi>, error out=w6:errorcluster)  [unwired: 3 in, 4 out]
  n185 = invoke class="VI" method="FP.Open"(reference=w8, error in=w6) -> (error out=w7:errorcluster)  [unwired: 3 in, 4 out]
  "error out" <- w7
  n186 = Delete(path (use dialog)=w12, error in=w7) -> ()  [unwired: 3 in, 3 out]
